vi "Read ADU Packet Master.vi"(8 "error in (no error)":errorcluster, 10 "Transaction ID":u16, 11 "TCP in":refnum<class "TCP.lvclass">) -> (0 "error out":errorcluster, 1 "Modbus Data Unit":T1={"function"=1, "Data"=[]} {"function" items=["Read Discrete Inputs"=2, "Read Coils"=1, "Write Single Coil"=5, "Write Multiple Coils"=15, "Read Input Register"=4, "Read Holding Registers"=3, "Write Single Register"=6, "Write Multiple Registers"=16, "Read/Write Multiple Registers"=23, "Mask Write Register"=22, "Read FIFO Queue"=24, "Read File Record"=20, "Write File Record"=21, "Read Exception Status"=7, "Diagnostic"=8, "Get Com Event Counter"=11, "Get Com Event Log"=12, "Report Slave ID"=17, "Read Device Identification"=43]; "Data" format="%.0x"}, 3 "TCP out":refnum<class "TCP.lvclass">, 5 "PDU Valid?":bool)   [LabVIEW 2021, in "NI_modbus_upd.lvlib"]
doc: "This uses the protocol layer to read a modbus packet off of the bus, wrapped in the IP transmission data unit."
uses:
  NI_modbus_upd.lvlib
  TCP/TCP.lvclass
  Ctl/MB Modbus Data Unit.ctl
  Modbus Data Unit (PDU)/Function.ctl
  TCP/TCP.lvclass/TCP.ctl
  <vilib>/Utility/error.llb/Clear Errors.vi
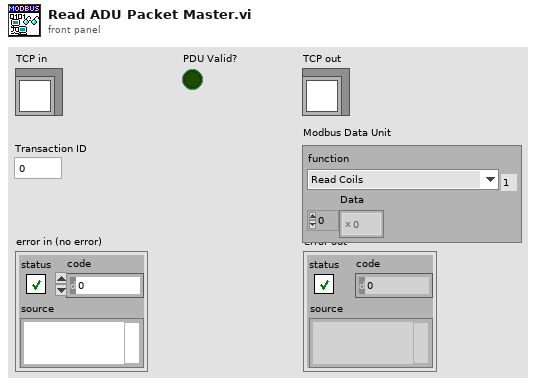
[diagram p1: front panel]
types:
  T1 = typedef "NI_modbus_upd.lvlib/MB Modbus Data Unit.ctl" = cluster{"function":T2, "Data":u8[]}
  T2 = typedef "NI_modbus_upd.lvlib/Function.ctl" = u8
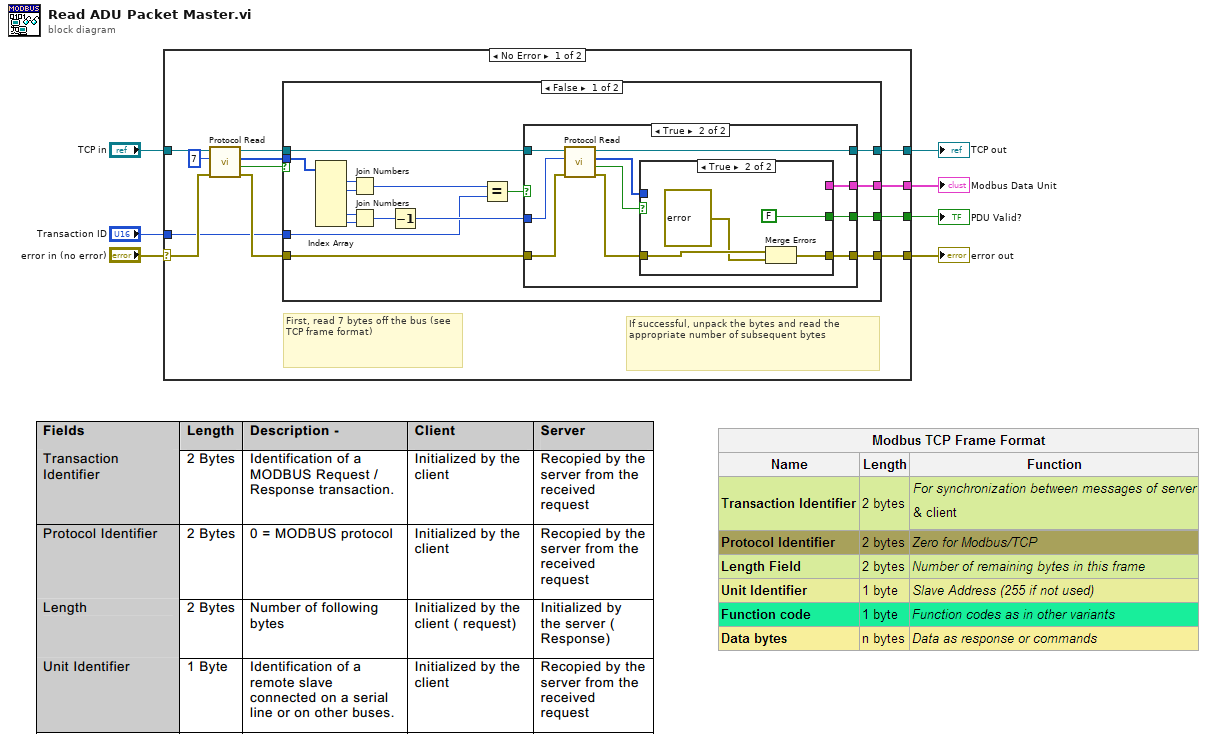
[diagram p0: block diagram]
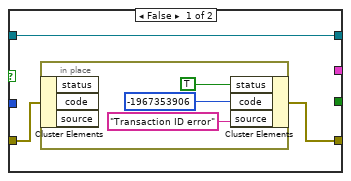
[diagram p2: hidden frame]
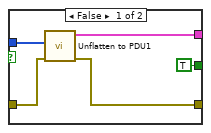
[diagram p3: hidden frame]
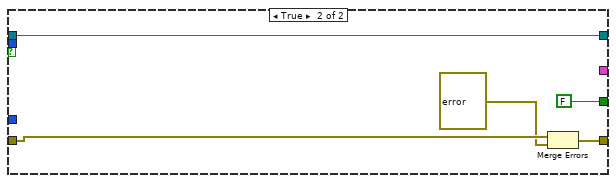
[diagram p4: hidden frame]
diagram:
  n1 = case shown="No Error" "error in (no error)" {
    selector: "error in (no error)" -> [w11 w67]
    tunnel: [w18 w67] -> w6
    tunnel: "TCP in" -> [w15 w66]
    tunnel: [w19 w66] -> w1
    tunnel: [w17 _] -> w2
    tunnel: [w16 _] -> w4
    tunnel: "Transaction ID" -> [w8 _]
    frame No Error {
      # "If successful, unpack the bytes and read the appropriate number of subsequent bytes"
      # "First, read 7 bytes off the bus (see TCP frame format)"
      n2 = call "Protocol Read.vi"("error in (no error)"=w11, "bytes to read"=7, "TCP in"=w15) -> ("error out"=w10:errorcluster, "timed out?"=w13:bool, "data"=w12:u8[], "TCP out"=w9:refnum<class "TCP.lvclass">)  [unwired: 5 in]
      n3 = case shown="False" w13 {
        tunnel: w12 -> [w20 _]
        tunnel: w9 -> [w22 w65]
        tunnel: [w21 w65] -> w19
        tunnel: w10 -> [w24 w63]
        tunnel: [w29 w64] -> w18
        tunnel: [w28 _] -> w17
        tunnel: [w27 FALSE] -> w16
        tunnel: w8 -> [w23 _]
        frame False {
          n4 = Index Array(array=w20) -> (element #1=w34:u8, element #2=w35:u8, element #5=w32:u8, element #6=w33:u8)  [unwired: 6 in, 2 out]
          n5 = Join Numbers(hi=w34, lo=w35) -> ((hi.lo)=w26:u16)
          n6 = Join Numbers(hi=w32, lo=w33) -> ((hi.lo)=w31:u16)
          n7 = Decrement(x=w31) -> (x-1=w30:u16)
          n8 = Equal?(x=w26, y=w23) -> (x = y?=w25:bool)
          n9 = case shown="True" w25 {
            tunnel: w30 -> [_ w47]
            tunnel: [w36 w51] -> w29
            tunnel: [_ w50] -> w28
            tunnel: [_ w49] -> w27
            tunnel: w24 -> [w37 w43]
            tunnel: w22 -> [w38 w48]
            tunnel: [w38 w44] -> w21
            frame False {
              n10 = in-place {
                n11 = in-place-cluster #1(w37) -> ()  [unwired: 3 out]
                n12 = in-place-cluster #1("status"=TRUE, "code"=-1967353906, "source"="Transaction ID error") -> (w36:errorcluster)
              }
            }
            frame True {
              n13 = call "Protocol Read.vi"("error in (no error)"=w43, "bytes to read"=w47, "TCP in"=w48) -> ("error out"=w42:errorcluster, "timed out?"=w46:bool, "data"=w45:u8[], "TCP out"=w44:refnum<class "TCP.lvclass">)  [unwired: 5 in]
              n14 = case shown="True" w46 {
                tunnel: [w52 w60] -> w51
                tunnel: [w55 _] -> w50
                tunnel: w45 -> [w54 _]
                tunnel: [TRUE FALSE] -> w49
                tunnel: w42 -> [w53 w58]
                frame False {
                  n15 = call "Unflatten to PDU1.vi"("error in (no error)"=w53, "Modbus data unit data"=w54) -> ("error out"=w52:errorcluster, "Modbus data unit out"=w55:T1)  [unwired: 8 in]
                }
                frame True {
                  n16 = Merge Errors(w58, errorcluster {"status"=TRUE, "code"=56, "source"="The network operation exceeded the user-specified or system time limit"} ("error in")) -> (w60:errorcluster)
                }
              }
            }
          }
        }
        frame True {
          n17 = Merge Errors(w63, errorcluster {"status"=TRUE, "code"=56, "source"="The network operation exceeded the user-specified or system time limit"} ("error in")) -> (w64:errorcluster)
        }
      }
    }
    frame Error {
    }
  }
  "error out" <- w6
  "PDU Valid?" <- w4
  "Modbus Data Unit" <- w2
  "TCP out" <- w1
